vi "Resolve Amplitude Settings.vi"(8 "Amplitude Unit (0: VPP)":i32(ring) items=["VPP", "VRMS", "DBM"], 11 "Amplitude (1 Vpp)":dbl=1.0) -> (3 "Resulting String":string)   [LabVIEW 2013, in "AWG.lvlib" / "Agilent 3352X Series.lvlib"]
doc: "Resolves the amplitude cluster to a setting string."
uses:
  Agilent 3352X Series.lvlib
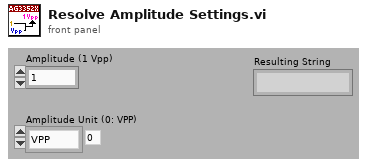
[diagram p1: front panel]
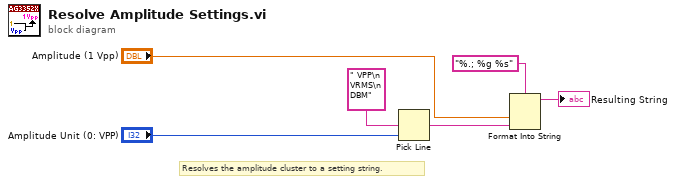
[diagram p0: block diagram]
diagram:
  # "Resolves the amplitude cluster to a setting string."
  n1 = Pick Line(multi-line string=" VPP\n VRMS\n DBM", line index="Amplitude Unit (0: VPP)") -> (output string=w4:string)  [unwired: 1 out]
  n2 = Format Into String(format string="%.; %g %s", "Amplitude (1 Vpp)", w4) -> (resulting string=→"Resulting String":string)  [unwired: 2 in, 1 out]
